vi "Create Messages.vi"(8 "error in (no error)":errorcluster, 10 "Ignore Previous Connections?":bool, 11 "Engine Data in":T2) -> (0 "error out":errorcluster, 1 "Connect Messages":T1[](array[typedef]), 2 "Disconnect Messages":T1[](array[typedef]), 3 "Engine Data out":T2)   [LabVIEW 2017, in "Routing and Faulting Engine.lvlib"]
uses:
  Routing and Faulting Engine.lvlib
  Engine Data.ctl
  Includes/CDMessaging.lvlibp/Producer/Abstract Producer/Abstract Producer.lvclass
  Shared/Compiled.Settings.ctl
  Shared/Communication Configuration.ctl
  Shared/Routing and Faulting Configuration.ctl
  Shared/Routing Channel Configuration.ctl
  Shared/Value-Connections Map.ctl
  Shared/Alias Mapping.ctl
  Shared/Compiled Connection.ctl
  Shared/FIFO Indices.ctl
  Device Inputs.ctl
  Device Outputs.ctl
  Producer Message.ctl
  Includes/CDMessaging.lvlibp/Message/Abstract Message/Abstract Message.lvclass
  3305a376-d4c0-444a-b726-8088d0367693.vi
  f117cfd3-3adc-40fc-b63f-36de5ebdde45.vi
  Shared/Get State Value Index.vi
  Shared/Convert State Value to Integer.vi
  Includes/CDMessaging.lvlibp/Switch/Switch Disconnect Message/Switch Disconnect Message.lvclass
  C:/Users/nitest/Documents/ni-official/niveristand-routing-and-faulting-custom-device/Includes/CDMessaging.lvlibp/Message/Abstract Request Message/Abstract Request Message.lvclass
  Includes/CDMessaging.lvlibp/Message/Abstract Request Message/Abstract Request Message.lvclass
  C:/Users/nitest/Documents/ni-official/niveristand-routing-and-faulting-custom-device/Includes/CDMessaging.lvlibp/Message/Abstract Message/Abstract Message.lvclass
  Includes/CDMessaging.lvlibp/Switch/Switch Connect Message/Switch Connect Message.lvclass
  <vilib>/Utility/error.llb/Error Cluster From Error Code.vi
  Shared/Routing and Faulting Shared.lvlib
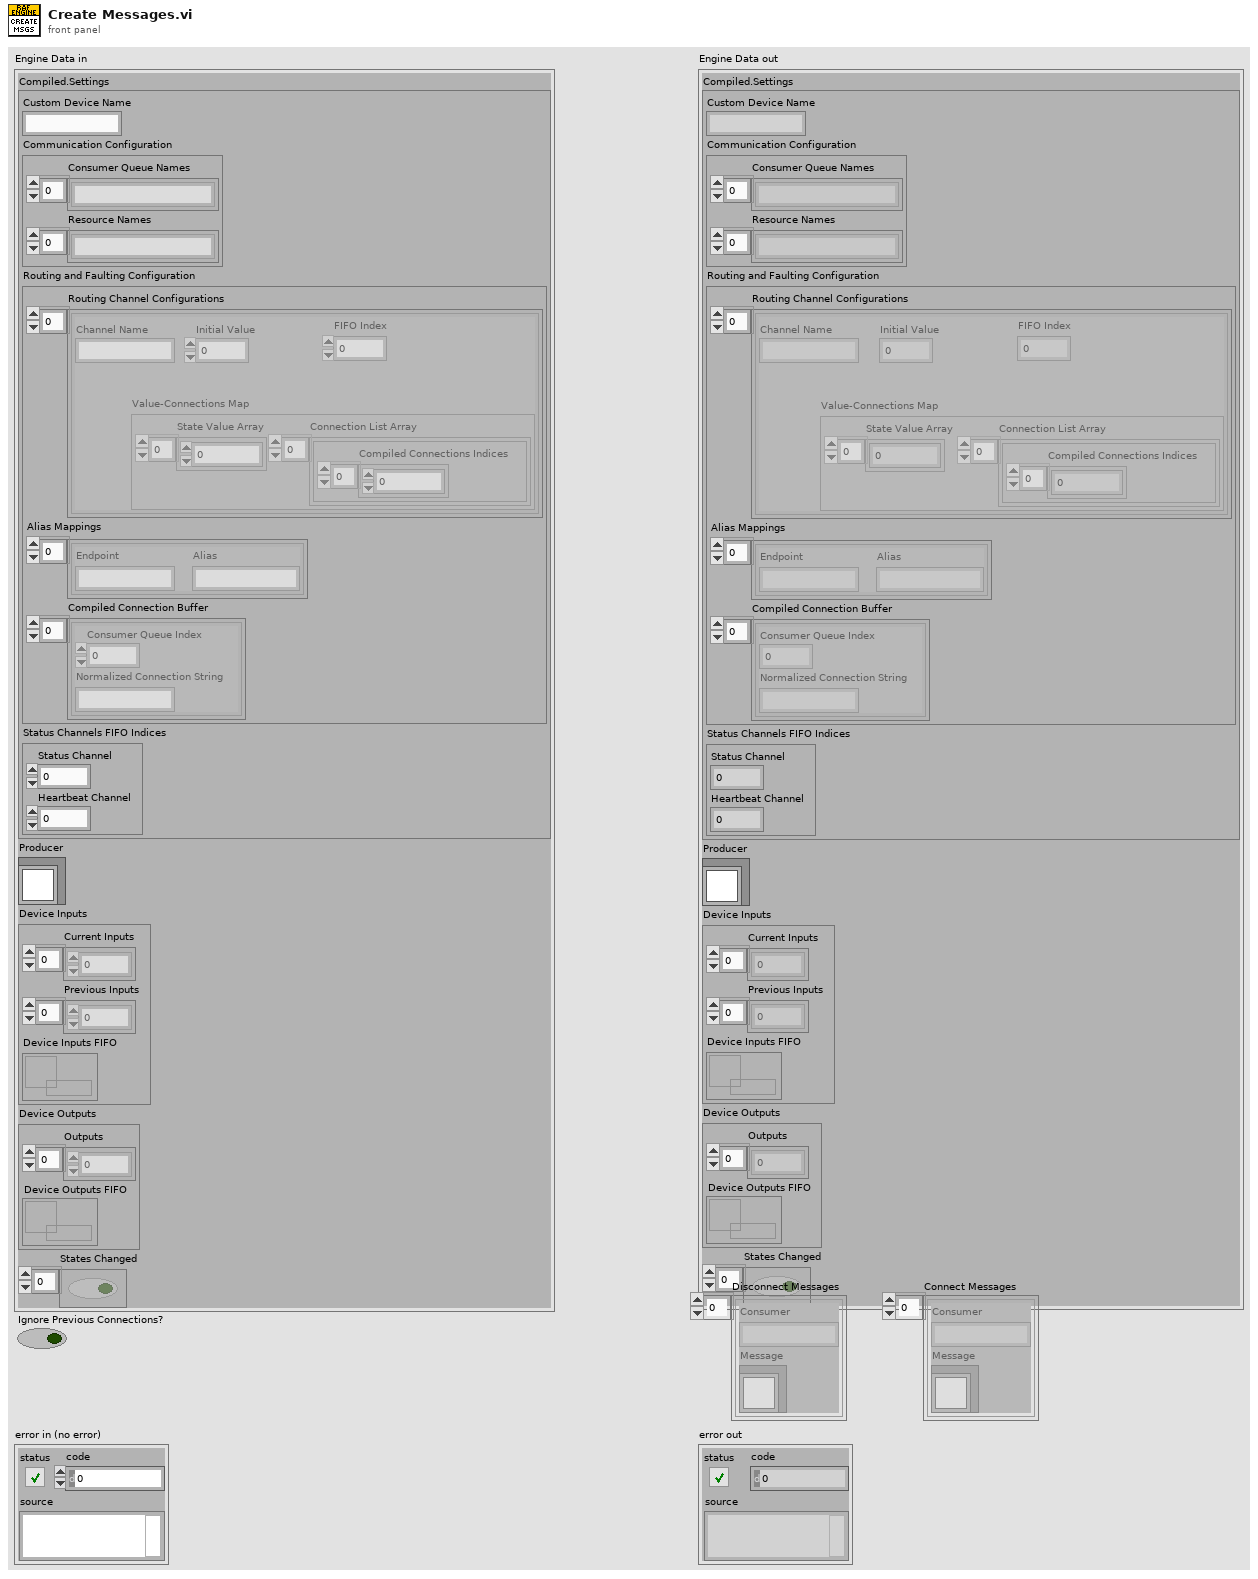
[diagram p1: front panel]
types:
  T1 = typedef "Routing and Faulting Engine.lvlib/Producer Message.ctl" = cluster{"Consumer":string, "Message":refnum<class "Abstract Message.lvclass">}
  T2 = typedef "Routing and Faulting Engine.lvlib/Engine Data.ctl" = cluster{"Compiled.Settings":T3, "Producer":refnum<class "Abstract Producer.lvclass">, "Device Inputs":T11, "Device Outputs":T12, "States Changed":bool[]}
  T3 = typedef "Routing and Faulting Shared.lvlib/Compiled.Settings.ctl" = cluster{"Custom Device Name":string, "Communication Configuration":T4, "Routing and Faulting Configuration":T5, "Status Channels FIFO Indices":T10}
  T4 = typedef "Routing and Faulting Shared.lvlib/Communication Configuration.ctl" = cluster{"Consumer Queue Names":string[], "Resource Names":string[]}
  T5 = typedef "Routing and Faulting Shared.lvlib/Routing and Faulting Configuration.ctl" = cluster{"Routing Channel Configurations":T6[], "Alias Mappings":T8[], "Compiled Connection Buffer":T9[]}
  T6 = typedef "Routing and Faulting Shared.lvlib/Routing Channel Configuration.ctl" = cluster{"Channel Name":string, "Initial Value":dbl, "FIFO Index":i32, "Value-Connections Map":T7}
  T7 = typedef "Routing and Faulting Shared.lvlib/Value-Connections Map.ctl" = cluster{"State Value Array":i32[], "Connection List Array":cluster{"Compiled Connections Indices":i32[]}[]}
  T8 = typedef "Routing and Faulting Shared.lvlib/Alias Mapping.ctl" = cluster{"Endpoint":string, "Alias":string}
  T9 = typedef "Routing and Faulting Shared.lvlib/Compiled Connection.ctl" = cluster{"Consumer Queue Index":i32, "Normalized Connection String":string}
  T10 = typedef "Routing and Faulting Shared.lvlib/FIFO Indices.ctl" = cluster{"Status Channel":i32, "Heartbeat Channel":i32}
  T11 = typedef "Routing and Faulting Engine.lvlib/Device Inputs.ctl" = cluster{"Current Inputs":dbl[], "Previous Inputs":dbl[], "Device Inputs FIFO":refnum<k33>}
  T12 = typedef "Routing and Faulting Engine.lvlib/Device Outputs.ctl" = cluster{"Outputs":dbl[], "Device Outputs FIFO":refnum<k33>}
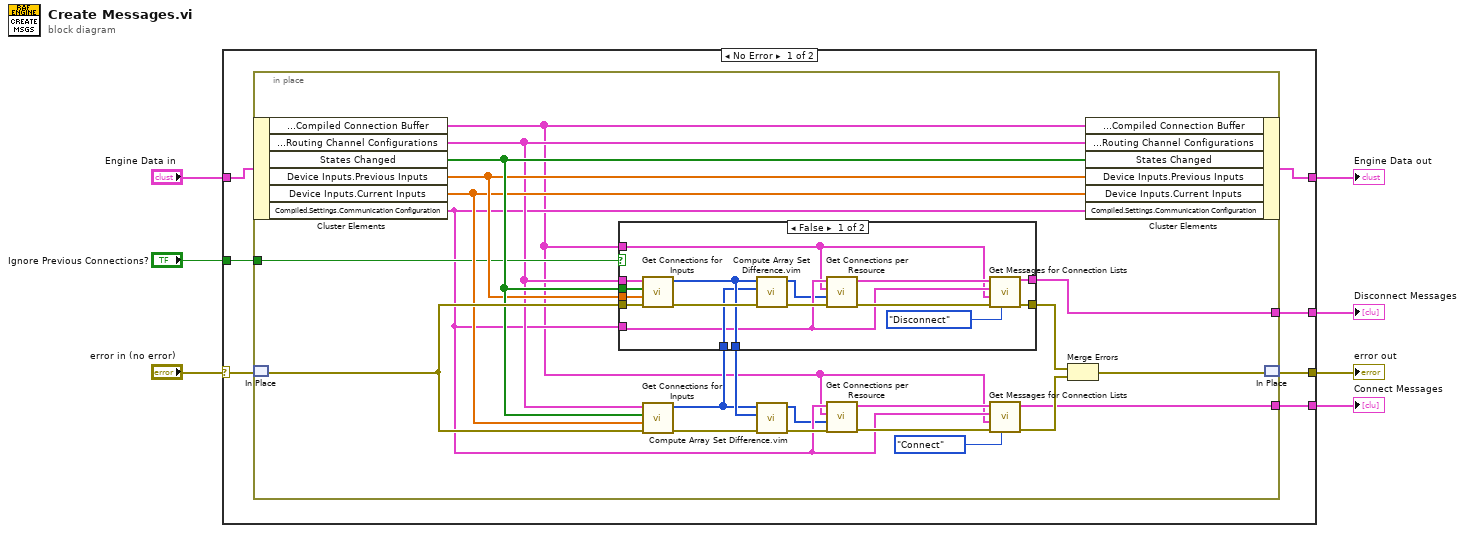
[diagram p0: block diagram]
diagram:
  n1 = case shown="No Error" "error in (no error)" {
    selector: "error in (no error)" -> [w14 w54]
    tunnel: "Engine Data in" -> [w10 w53]
    tunnel: [w13 w54] -> w5
    tunnel: [w12 w53] -> w4
    tunnel: [w11 _] -> w3
    tunnel: [w9 _] -> w2
    tunnel: "Ignore Previous Connections?" -> [w8 _]
    frame No Error {
      n2 = in-place {
        in-place-border: [w35] -> w11
        in-place-border: [w21] -> w9
        in-place-border: w8 -> [w20]
        n3 = in-place-cluster #1(w10) -> ("Compiled.Settings.Routing and Faulting Configuration.Compiled Connection Buffer"=w16:T9[], "Compiled.Settings.Routing and Faulting Configuration.Routing Channel Configurations"=w19:T6[], "States Changed"=w33:bool[], "Device Inputs.Previous Inputs"=w26:dbl[], "Device Inputs.Current Inputs"=w25:dbl[], "Compiled.Settings.Communication Configuration"=w18:T4)
        n4 = in-place-match #2(w14) -> (w34:errorcluster)
        n5 = call "Get Connections for Inputs.vi"("error in (no error)"=w34, "Inputs"=w25, "States Changed"=w33, "Routing Channel Configurations"=w19) -> ("error out"=w30:errorcluster, "Compiled Connections Indices"=w31:i32[])  [unwired: 6 in]
        n6 = case shown="False" w20 {
          tunnel: [w50 _] -> w35
          tunnel: w34 -> [w47 w52]
          tunnel: w19 -> [w46 _]
          tunnel: w33 -> [w45 _]
          tunnel: [w44 _] -> w32
          tunnel: w31 -> [w43 _]
          tunnel: w26 -> [w41 _]
          tunnel: [w40 w52] -> w24
          tunnel: w18 -> [w39 _]
          tunnel: w16 -> [w37 _]
          frame False {
            n7 = call "Get Connections for Inputs.vi"("error in (no error)"=w47, "Inputs"=w41, "States Changed"=w45, "Routing Channel Configurations"=w46) -> ("error out"=w51:errorcluster, "Compiled Connections Indices"=w44:i32[])  [unwired: 6 in]
            n8 = call "Compute Array Set Difference.vim"("error in (no error)"=w51, "B"=w43, "A"=w44) -> ("error out"=w42:errorcluster, "A - B"=w36:i32[])  [unwired: 7 in]
            n9 = call "Get Connections per Resource.vi"("error in (no error)"=w42, "Compiled Connections Indices"=w36, "Compiled Connection Buffer"=w37, "Communication Configuration"=w39) -> ("error out"=w48:errorcluster, "Connection Lists for each Resource"=w49:cluster{"Indices":i32[]}[])  [unwired: 6 in]
            n10 = call "Get Messages for Connection Lists.vi"("Message Type"=enum16{"Connect", "Disconnect"}."Disconnect", "error in (no error)"=w48, "Compiled Connection Buffer"=w37, "Communication Configuration"=w39, "Connection Lists for each Resource"=w49) -> ("error out"=w40:errorcluster, "Messages"=w50:T1[])  [unwired: 5 in]
          }
          frame True {
          }
        }
        n11 = call "Compute Array Set Difference.vim"("error in (no error)"=w30, "B"=w32, "A"=w31) -> ("error out"=w27:errorcluster, "A - B"=w17:i32[])  [unwired: 7 in]
        n12 = call "Get Connections per Resource.vi"("error in (no error)"=w27, "Compiled Connections Indices"=w17, "Compiled Connection Buffer"=w16, "Communication Configuration"=w18) -> ("error out"=w29:errorcluster, "Connection Lists for each Resource"=w28:cluster{"Indices":i32[]}[])  [unwired: 6 in]
        n13 = call "Get Messages for Connection Lists.vi"("Message Type"=enum16{"Connect", "Disconnect"}."Connect", "error in (no error)"=w29, "Compiled Connection Buffer"=w16, "Communication Configuration"=w18, "Connection Lists for each Resource"=w28) -> ("error out"=w23:errorcluster, "Messages"=w21:T1[])  [unwired: 5 in]
        n14 = Merge Errors(w24, w23) -> (w22:errorcluster)
        n15 = in-place-cluster #1("Compiled.Settings.Routing and Faulting Configuration.Compiled Connection Buffer"=w16, "Compiled.Settings.Routing and Faulting Configuration.Routing Channel Configurations"=w19, "States Changed"=w33, "Device Inputs.Previous Inputs"=w26, "Device Inputs.Current Inputs"=w25, "Compiled.Settings.Communication Configuration"=w18) -> (w12:T2)
        n16 = in-place-match #2(w22) -> (w13:errorcluster)
      }
    }
    frame Error {
    }
  }
  "Engine Data out" <- w4
  "error out" <- w5
  "Disconnect Messages" <- w3
  "Connect Messages" <- w2
